vi "ex8_traffic light.vi"() -> ()   [LabVIEW 2018]
panel:
  in  "Cross?":bool
  out "Pedestrian 4":bool
  out "Time remaining":dbl caption="Numeric"
  in  "stop":bool
  out "Green 3":bool
  out "Yellow 2":bool
  out "Red":bool
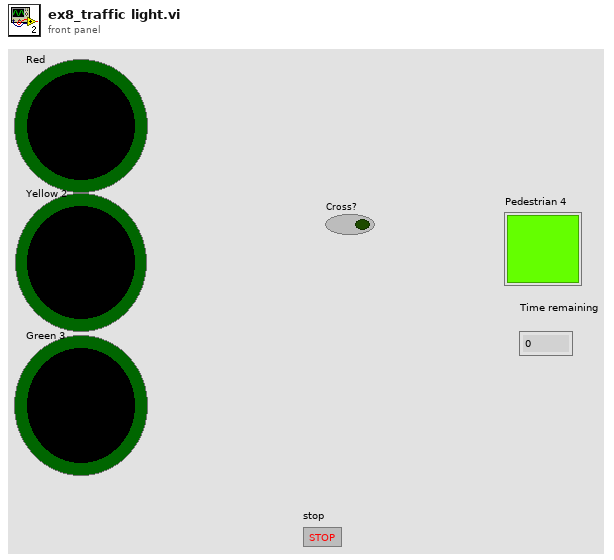
[diagram p1: front panel]
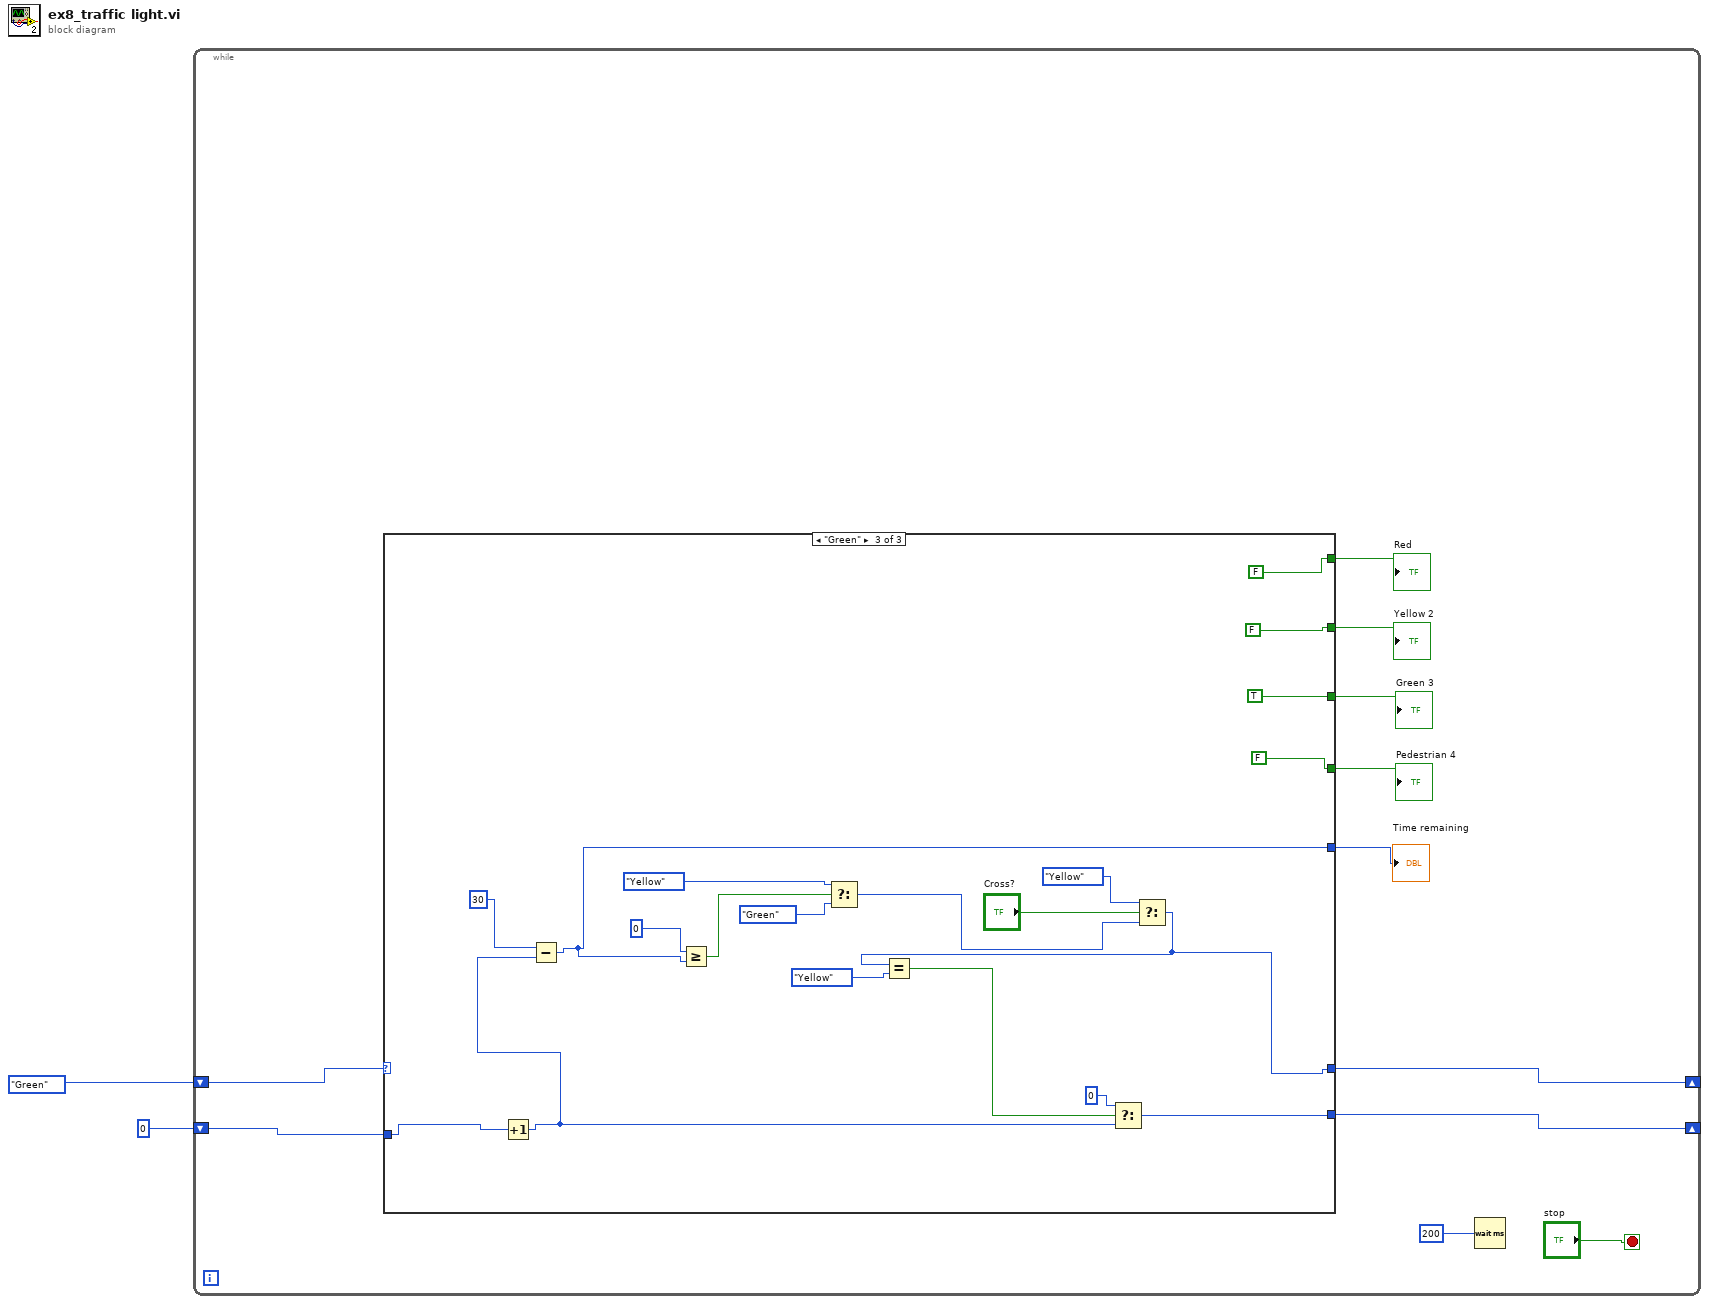
[diagram p0: block diagram]
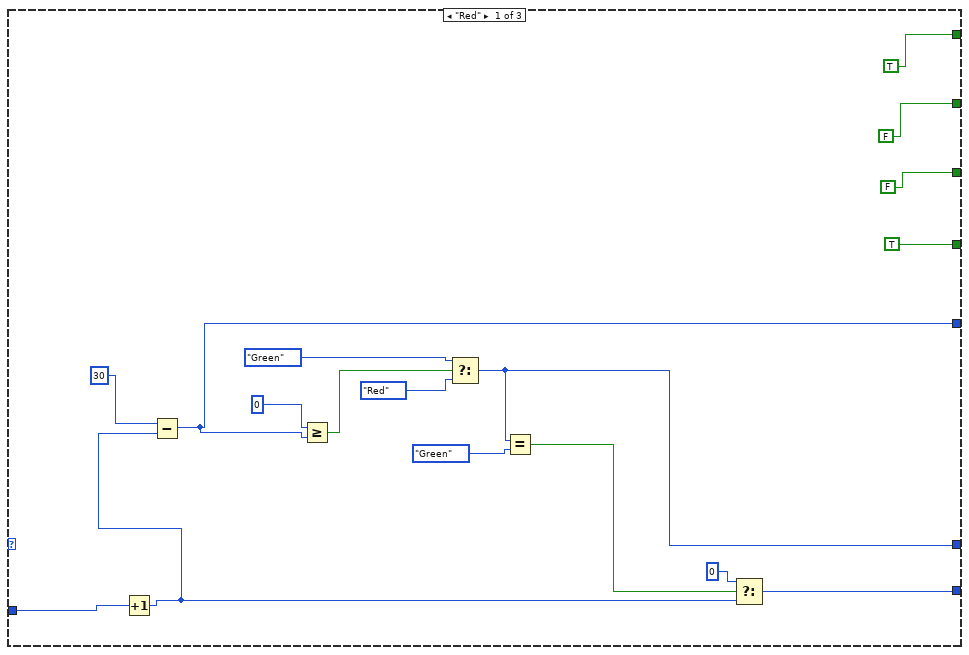
[diagram p2: hidden frame]
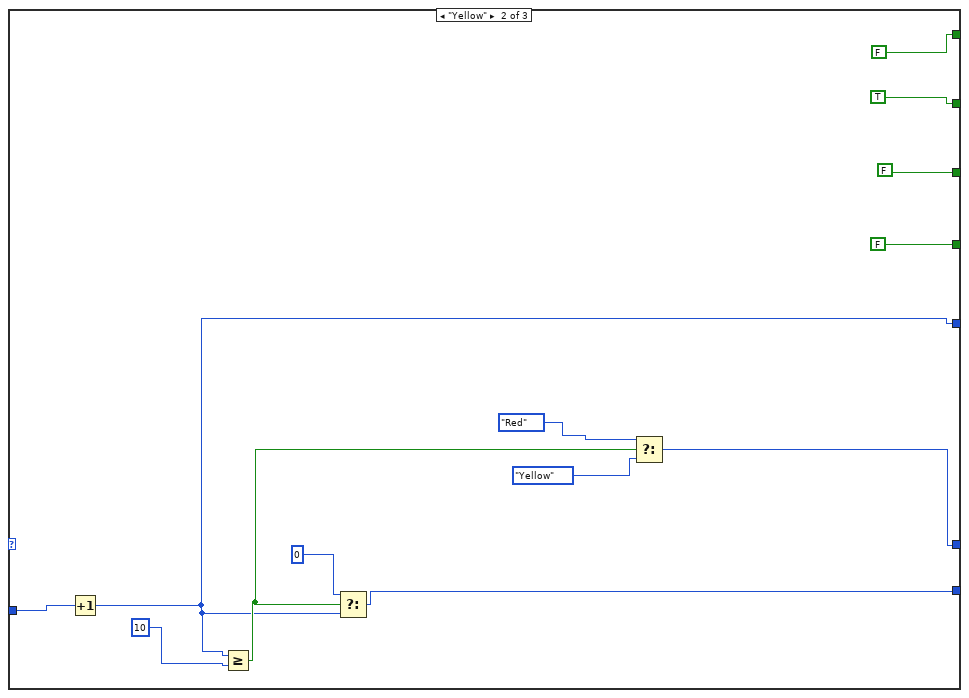
[diagram p3: hidden frame]
diagram:
  n1 = while {
    shift-right: [w8] -> _
    shift-left: enum16{"Red", "Yellow", "Green"}."Green" -> [w12]
    shift-right: [w9] -> _
    shift-left: 0 -> [w10]
    stop <- "stop" stop-if-true
    n2 = case shown="\"Green\"" w12 {
      tunnel: w10 -> [w30 w43 w50]
      tunnel: [w27 w38 w48] -> w9
      tunnel: [w26 w39 w44] -> w8
      tunnel: [TRUE FALSE FALSE] -> w7
      tunnel: [FALSE TRUE FALSE] -> w6
      tunnel: [FALSE FALSE TRUE] -> w5
      tunnel: [TRUE FALSE FALSE] -> w4
      tunnel: [w14 w31 w49] -> w3
      frame "Red" {
        n3 = Increment(x=w30) -> (x+1=w16:i32)
        n4 = Subtract(x=30, y=w16) -> (x-y=w14:i32)
        n5 = Greater Or Equal?(x=0, y=w14) -> (x >= y?=w18:bool)
        n6 = Select(t=enum16{"Red", "Yellow", "Green"}."Green", s=w18, f=enum16{"Red", "Yellow", "Green"}."Red") -> (s? t:f=w26:enum16{"Red", "Yellow", "Green"})
        n7 = Equal?(x=w26, y=enum16{"Red", "Yellow", "Green"}."Green") -> (x = y?=w29:bool)
        n8 = Select(t=0, s=w29, f=w16) -> (s? t:f=w27:i32)
      }
      frame "Yellow" {
        n9 = Increment(x=w43) -> (x+1=w31:i32)
        n10 = Greater Or Equal?(x=w31, y=10 ("t")) -> (x >= y?=w32:bool)
        n11 = Select(t=0, s=w32, f=w31) -> (s? t:f=w38:i32)
        n12 = Select(t=enum16{"Red", "Yellow", "Green"}."Red", s=w32, f=enum16{"Red", "Yellow", "Green"}."Yellow") -> (s? t:f=w39:enum16{"Red", "Yellow", "Green"})
      }
      frame "Green" {
        n13 = Increment(x=w50) -> (x+1=w52:i32)
        n14 = Subtract(x=30, y=w52) -> (x-y=w49:i32)
        n15 = Greater Or Equal?(x=0, y=w49) -> (x >= y?=w54:bool)
        n16 = Select(t=enum16{"Red", "Yellow", "Green"}."Yellow", s=w54, f=enum16{"Red", "Yellow", "Green"}."Green") -> (s? t:f=w45:enum16{"Red", "Yellow", "Green"})
        n17 = Select(t=enum16{"Red", "Yellow", "Green"}."Yellow", s="Cross?", f=w45) -> (s? t:f=w44:enum16{"Red", "Yellow", "Green"})
        n18 = Equal?(x=w44, y=enum16{"Red", "Yellow", "Green"}."Yellow") -> (x = y?=w59:bool)
        n19 = Select(t=0, s=w59, f=w52) -> (s? t:f=w48:i32)
      }
    }
    "Green 3" <- w5
    "Yellow 2" <- w6
    "Red" <- w7
    "Pedestrian 4" <- w4
    "Time remaining" <- w3
    n20 = Wait (ms)(milliseconds to wait=u32 200 ("millisecond timer value")) -> ()  [unwired: 1 out]
  }
